vi "ConfigureDlg.vi"(8 "error in (no error)":errorcluster, 11 "PmuBase in":refnum<class "PmuBase.lvclass">) -> (0 "error out":errorcluster, 2 "Changed":bool, 3 "PmuBase out":refnum<class "PmuBase.lvclass">)   [LabVIEW 2018, in "SensorPlugins.lvlib" / "PmuBase.lvclass"]
uses:
  PmuBase.lvclass
  C:/Program Files/National Instruments/LabVIEW 2018/user.lib/NIST/BaseClasses/BasePlugin_class/BasePlugin.lvclass
  Typedef/PmuConfig.ctl
  Typedef/ePhases.ctl
  PmuBase.lvclass/PmuBase.ctl
  <userlib>/NIST/BaseClasses/BasePlugin_class/BasePlugin.lvclass/BasePlugin.ctl
  Accessors/Read PhaseArray.vi
  Accessors/Read PmuConfig.vi
  Accessors/Write PmuConfig.vi
  Accessors/Write PhaseArray.vi
  <userlib>/NIST/BaseClasses/BasePlugin_class/Accessors/Read PluginIniFilePath.vi
  <userlib>/NIST/BaseClasses/BasePlugin_class/Accessors/Write PluginIniFilePath.vi
  <vilib>/Utility/config.llb/NI_LVConfig.lvlib
  <userlib>/NIST/NISTErrorLib/NISTErrorLib.lvlib
panel:
  in  "btnCancel":bool
  in  "btnSaveAs":bool
  in  "BtnDone":bool
  in  "PhaseArray":T1[](array[typedef])=[enum."VA", enum."VB", enum."VC", enum."V+", enum."IA", enum."IB", enum."IC", enum."I+"]
  in  "PmuConfig":T2={"Class"=enum."M", "Fs"=60, "F0"=60, "FSamp"=60, "SettlingTime"=0.0, "T0"=0.0}
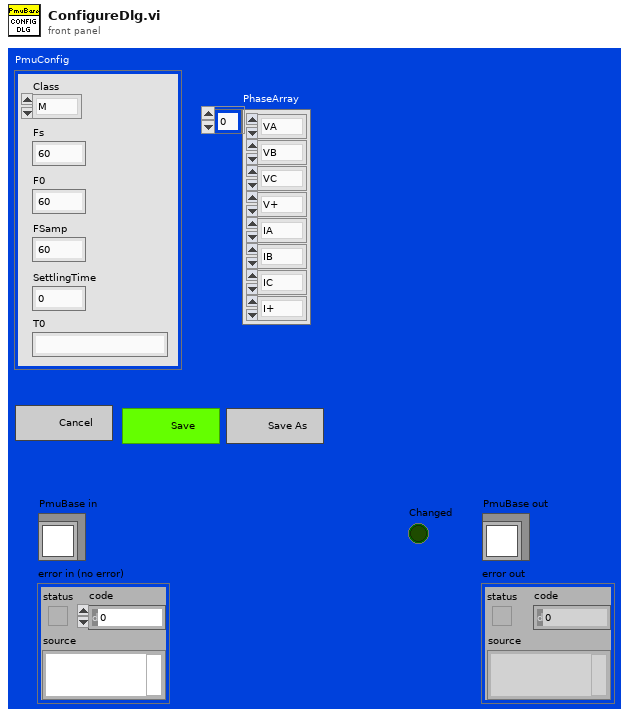
[diagram p1: front panel]
types:
  T1 = typedef "SensorPlugins.lvlib/PmuBase.lvclass/ePhases.ctl" = enum16{"VA", "VB", "VC", "V+", "IA", "IB", "IC", "I+", "none"}
  T2 = typedef "SensorPlugins.lvlib/PmuBase.lvclass/PmuConfig.ctl" = cluster{"Class":enum16{"M", "P"}, "Fs":i32, "F0":i32, "FSamp":i32, "SettlingTime":dbl, "T0":ext}
  T3 = enum32{"Invalid", "Standard", "Closed", "Hidden", "Minimized", "Maximized"}
  T4 = enum32{"Invalid", "Default", "Floating", "Floating/Auto-Hide", "Modal"}
  T5 = enum8{"Enabled", "Disabled", "Disabled and Grayed Out"}
  T6 = typedef "NI_LVConfig.lvlib/Config Data RefNum.ctl" = refnum<k1>
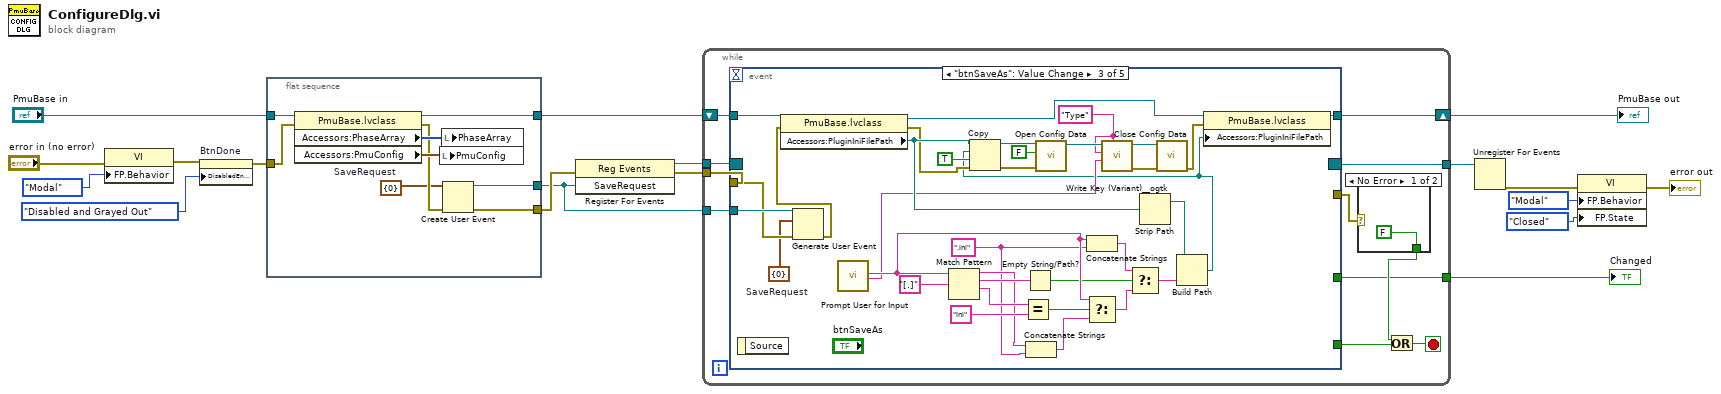
[diagram p0: block diagram]
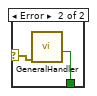
[diagram p2: hidden frame]
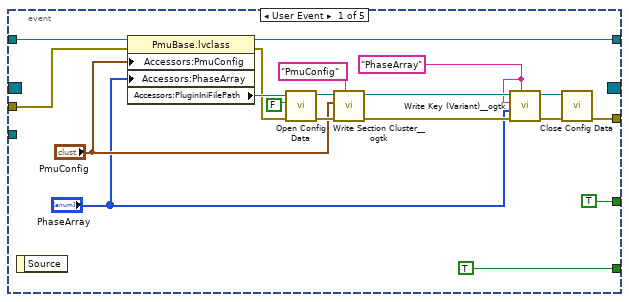
[diagram p3: hidden frame]
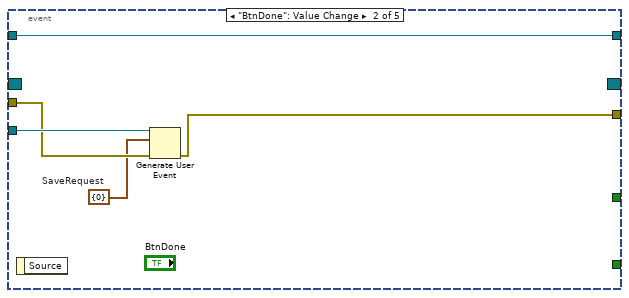
[diagram p4: hidden frame]
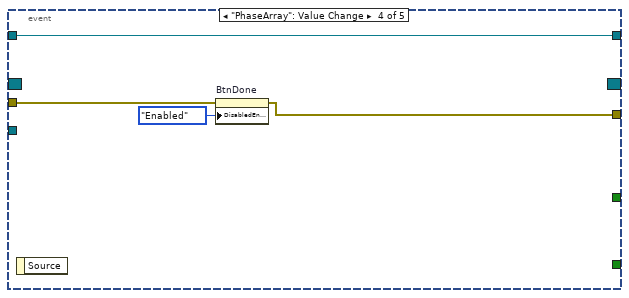
[diagram p5: hidden frame]
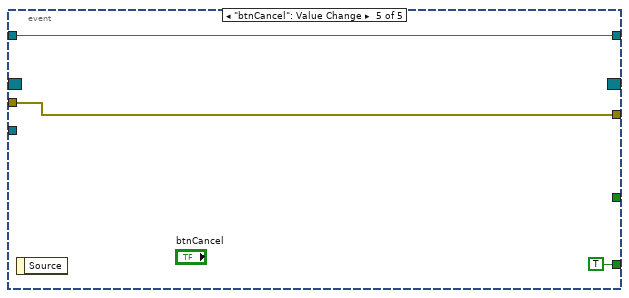
[diagram p6: hidden frame]
diagram:
  n1 = property class="VI"(error in="error in (no error)", "FP.Behavior"=T4."Modal" ("Front Panel Window:Behavior")) -> (error out=w16:errorcluster)  [unwired: 1 in, 1 out]
  n2 = property on="BtnDone" class="Bool"(error in=w16, "DisabledEnum"=T5."Disabled and Grayed Out" ("Disabled")) -> (error out=w13:errorcluster)  [unwired: 1 in, 1 out]
  n3 = flat-sequence {
    tunnel: "PmuBase in" -> [w27]
    tunnel: w13 -> [w26]
    tunnel: [w22] -> w11
    tunnel: [w21] -> w8
    tunnel: [w20] -> w12
    frame #0 {
      w19 = cluster{"Num":i32} {"Num"=0}  # SaveRequest
      n4 = property class="PmuBase.lvclass"(reference=w27, error in=w26) -> (reference out=w22:refnum<class "PmuBase.lvclass">, error out=w23:errorcluster, "Accessors:PhaseArray"=w25:T1[], "Accessors:PmuConfig"=w24:T2)
      n5 = local write "PmuConfig"(w24) -> ()
      n6 = local write "PhaseArray"(w25) -> ()
      n7 = Create User Event(user event datatype=w19, error in=w23) -> (user event=w21:refnum<user-event>, error out=w20:errorcluster)
    }
  }
  n8 = register-events(error in=w12, w8) -> (reference out=w10:refnum<event-registration>, error out=w9:errorcluster)  [unwired: 1 in]
  n9 = while {
    shift-right: [w35] -> w1
    shift-left: w11 -> [w37]
    tunnel: w10 -> [w38]
    tunnel: w9 -> [w36]
    tunnel: w8 -> [w29]
    tunnel: [w34] -> w7
    tunnel: [w28] -> w6
    stop <- w32 stop-if-true
    n10 = event shown="[2] \"btnSaveAs\": Value Change" {
      selector: w38 -> [_ _ _ _ _]
      dyn-events: [_ _ _ _ _] -> w34
      timeout: _ -> [_ _ _ _ _]
      tunnel: w37 -> [w60 w62 w83 w100 w104]
      tunnel: w36 -> [w59 w64 w84 w103 w105]
      tunnel: [w45 w63 _ w101 w105] -> w33
      tunnel: [w44 w62 w70 w100 w104] -> w35
      tunnel: [TRUE _ _ _ TRUE] -> w30
      tunnel: w29 -> [_ w65 w85 _ _]
      tunnel: [TRUE _ _ _ _] -> w28
      event User Event {
        w48 = "PhaseArray" ("section")
        n11 = event-data() -> ()  [unwired: 1 in, 1 out]
        n12 = property class="PmuBase.lvclass"(reference=w60, error in=w59, "Accessors:PmuConfig"="PmuConfig", "Accessors:PhaseArray"="PhaseArray") -> (reference out=w44:refnum<class "PmuBase.lvclass">, error out=w56:errorcluster, "Accessors:PluginIniFilePath"=w58:path)
        n13 = call <vilib>:"Open Config Data.vi"("error in (no error)"=w56, "create file if necessary (T)"=FALSE, "configuration file path"=w58) -> ("error out"=w55:errorcluster, "refnum"=w54:T6)  [unwired: 6 in, 1 out]
        n14 = call <userlib>:"Write Section Cluster__ogtk.vi"("section (optional)"="PmuConfig", "error in (no error)"=w55, "Section Formatted Cluster"="PmuConfig", "refnum"=w54) -> ("error out"=w51:errorcluster, "dup refnum"=w50:T6)  [unwired: 6 in]
        n15 = call <userlib>:"Write Key (Variant)__ogtk.vi"("section"=w48, "error in (no error)"=w51, "key-value"="PhaseArray", "key (optional)"=w48, "refnum"=w50) -> ("error out"=w47:errorcluster, "refnum out"=w46:T6)  [unwired: 5 in]
        n16 = call <vilib>:"Close Config Data.vi"("error in (no error)"=w47, "refnum"=w46) -> ("error out"=w45:errorcluster)  [unwired: 8 in, 1 out]
      }
      event "BtnDone": Value Change {
        w61 = cluster{"Num":i32} {"Num"=0}  # SaveRequest
        n17 = event-data() -> ()  [unwired: 1 in, 1 out]
        n18 = Generate User Event(user event=w65, event data cluster=w61, error in=w64) -> (error out=w63:errorcluster)  [unwired: 1 in, 1 out]
      }
      event "btnSaveAs": Value Change {
        w66 = cluster{"Num":i32} {"Num"=0}  # SaveRequest
        w74 = "Type" ("section")
        w88 = ".ini" ("string")
        n19 = event-data() -> ()  [unwired: 1 in, 1 out]
        n20 = Generate User Event(user event=w85, event data cluster=w66, error in=w84) -> (error out=w82:errorcluster)  [unwired: 1 in, 1 out]
        n21 = property class="PmuBase.lvclass"(reference=w83, error in=w82) -> (reference out=w69:refnum<class "PmuBase.lvclass">, error out=w79:errorcluster, "Accessors:PluginIniFilePath"=w81:path)
        n22 = call "Prompt User for Input"() -> ("File Name"=w99:string, "PluginType Name"=w73:string)  [unwired: 16 in, 2 out]
        n23 = Match Pattern(string=w99, regular expression="[.]" ("string")) -> (before substring=w89:string, match substring=w92:string, after substring=w91:string)  [unwired: 1 in, 1 out]
        n24 = Equal?(x=w91, y="ini" ("string")) -> (x = y?=w94:bool)
        n25 = Empty String/Path?(string/path=w92) -> (empty?=w95:bool)
        n26 = Concatenate Strings(w89, w88) -> (w87:string)
        n27 = Concatenate Strings(w99, w88) -> (w97:string)
        n28 = Select(t=w99, s=w94, f=w87) -> (s? t:f=w96:string)
        n29 = Select(t=w97, s=w95, f=w96) -> (s? t:f=w98:string)
        n30 = Strip Path(path=w81) -> (stripped path=w86:path)  [unwired: 1 out]
        n31 = Build Path(base path=w86, name or relative path=w98) -> (appended path=w67:path)
        n32 = Copy(8:w79, 9:TRUE ("overwrite (F)"), 10:w67, 11:w81) -> (0:w76:errorcluster, 3:w78:path)  [unwired: 1 in, 1 out]
        n33 = call <vilib>:"Open Config Data.vi"("error in (no error)"=w76, "create file if necessary (T)"=FALSE, "configuration file path"=w78) -> ("refnum"=w75:T6)  [unwired: 6 in, 2 out]
        n34 = call <userlib>:"Write Key (Variant)__ogtk.vi"("section"=w74, "key-value"=w73, "key (optional)"=w74, "refnum"=w75) -> ("error out"=w72:errorcluster, "refnum out"=w71:T6)  [unwired: 6 in]
        n35 = call <vilib>:"Close Config Data.vi"("error in (no error)"=w72, "refnum"=w71) -> ("error out"=w68:errorcluster)  [unwired: 8 in, 1 out]
        n36 = property class="PmuBase.lvclass"(reference=w69, error in=w68, "Accessors:PluginIniFilePath"=w67) -> (reference out=w70:refnum<class "PmuBase.lvclass">)  [unwired: 1 out]
      }
      event "PhaseArray": Value Change {
        n37 = event-data() -> ()  [unwired: 1 in, 1 out]
        n38 = property on="BtnDone" class="Bool"(error in=w103, "DisabledEnum"=T5."Enabled" ("Disabled")) -> (error out=w101:errorcluster)  [unwired: 1 in, 1 out]
      }
      event "btnCancel": Value Change {
        n39 = event-data() -> ()  [unwired: 1 in, 1 out]
      }
    }
    n40 = case shown="No Error" w33 {
      selector: w33 -> [_ w41]
      tunnel: [FALSE w40] -> w31
      frame No Error {
      }
      frame Error {
        n41 = call <userlib>:"GeneralHandler.vi"("error in (no error)"=w41) -> ("Stop"=w40:bool)  [unwired: 6 in, 4 out]
      }
    }
    n42 = Or(x=w31, y=w30) -> (x .or. y?=w32:bool)
  }
  "PmuBase out" <- w1
  "Changed" <- w6
  n43 = Unregister For Events(event registration refnum=w7) -> (error out=w3:errorcluster)  [unwired: 1 in]
  n44 = property class="VI"(error in=w3, "FP.Behavior"=T4."Modal" ("Front Panel Window:Behavior"), "FP.State"=T3."Closed" ("Front Panel Window:State")) -> (error out=→"error out":errorcluster)  [unwired: 1 in, 1 out]
